vi "Motion@AddPallet__Parameter.vi"(1 "ParamterIn":string) -> (0 "ParamterOut":string)   [LabVIEW 2020]
panel:
  in  "AXIS":string(combo)
  in  "PointName":string(combo)
  in  "Speed":string(combo)
  in  "MotorName":string(combo)
  in  "Confirm":bool
  # "Motion@AddPallet $Motor,$Speed,$Point(@AXIS)\nExample:  $Point@XY will move XY only\n               $Point@XYZ(5) will move XYZ and Z will replace by 5"
  # "@"
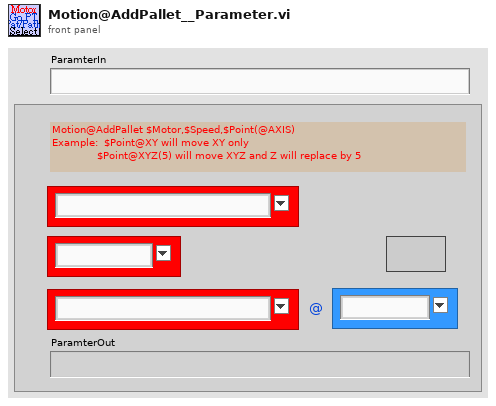
[diagram p1: front panel]
types:
  T1 = enum16{"Get", "UpdatePointS", "Init", "UpdateIndex", "GetCurrent&Index+1", "GetWithIndex", "ChkLast", "GetCurrent"}
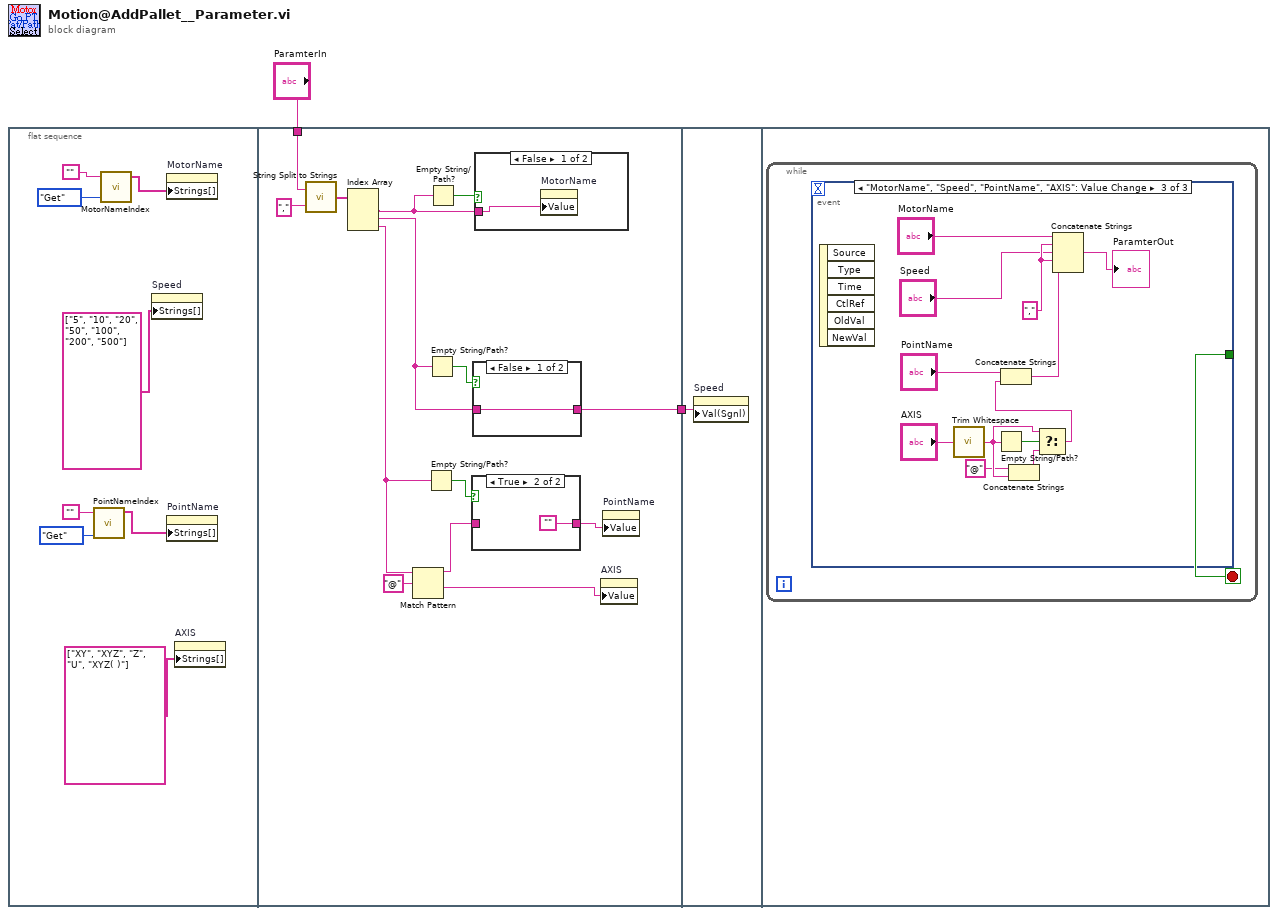
[diagram p0: block diagram]
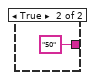
[diagram p3: hidden frame]
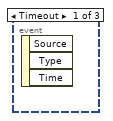
[diagram p5: hidden frame]
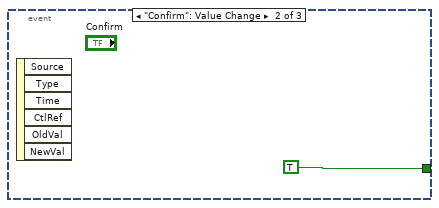
[diagram p6: hidden frame]
diagram:
  n1 = flat-sequence {
    tunnel: "ParamterIn" -> [w20]
    tunnel: [w16] -> w1
    tunnel: w1 -> [w30]
    frame #0 {
      n2 = call "PointNameIndex.vi"("OP"=T1."Get", "PointName"="") -> ("PointNameList"=w4:string[])  [unwired: 4 in, 5 out]
      n3 = call "MotorNameIndex.vi"("OP"=enum16{"Get", "Update", "Init"}."Get", "MotorName"="") -> ("MotorList"=w8:string[])  [unwired: 1 in, 2 out]
      n4 = property on="Speed" class="CmbBox"("Strings[]"=string[] ["5", "10", "20", "50", "100", "200", "500"] ("Strings []")) -> ()  [unwired: 2 in, 2 out]
      n5 = property on="MotorName" class="CmbBox"("Strings[]"=w8) -> ()  [unwired: 2 in, 2 out]
      n6 = property on="PointName" class="CmbBox"("Strings[]"=w4) -> ()  [unwired: 2 in, 2 out]
      n7 = property on="AXIS" class="CmbBox"("Strings[]"=string[] ["XY", "XYZ", "Z", "U", "XYZ( )"] ("Strings []")) -> ()  [unwired: 2 in, 2 out]
    }
    frame #1 {
      n8 = call "String Split to Strings.vi"("search string/char (-)"=",", "String"=w20) -> ("Array"=w22:string[])
      n9 = Index Array(array=w22) -> (element #1=w19:string, element #2=w18:string, element #3=w14:string)  [unwired: 3 in]
      n10 = Match Pattern(string=w14, regular expression="@") -> (before substring=w11:string, after substring=w12:string)  [unwired: 1 in, 2 out]
      n11 = Empty String/Path?(string/path=w14) -> (empty?=w17:bool)
      n12 = Empty String/Path?(string/path=w18) -> (empty?=w23:bool)
      n13 = Empty String/Path?(string/path=w19) -> (empty?=w24:bool)
      n14 = case shown="True" w17 {
        tunnel: [w25 ""] -> w15
        tunnel: w11 -> [w25 _]
        frame False {
        }
        frame True {
        }
      }
      n15 = case shown="False" w23 {
        tunnel: [w27 "50" ("ParamterIn")] -> w16
        tunnel: w18 -> [w27 _]
        frame False {
        }
        frame True {
        }
      }
      n16 = case shown="False" w24 {
        tunnel: w19 -> [w29 _]
        frame False {
          n17 = property on="MotorName" class="CmbBox"("Value"=w29) -> ()  [unwired: 2 in, 2 out]
        }
        frame True {
        }
      }
      n18 = property on="AXIS" class="CmbBox"("Value"=w12) -> ()  [unwired: 2 in, 2 out]
      n19 = property on="PointName" class="CmbBox"("Value"=w15) -> ()  [unwired: 2 in, 2 out]
    }
    frame #2 {
      n20 = property on="Speed" class="CmbBox"("Val(Sgnl)"=w30) -> ()  [unwired: 2 in, 2 out]
    }
    frame #3 {
      n21 = while {
        stop <- w31 stop-if-true
        n22 = event shown="[2] \"MotorName\", \"Speed\", \"PointName\", \"AXIS\": Value Change" {
          selector: _ -> [_ _ _]
          dyn-events: _ -> [_ _ _]
          timeout: _ -> [_ _ _]
          tunnel: [_ TRUE _] -> w31
          event Timeout {
            n23 = event-data() -> ()  [unwired: 1 in, 3 out]
          }
          event "Confirm": Value Change {
            n24 = event-data() -> ()  [unwired: 1 in, 6 out]
          }
          event "MotorName", "Speed", "PointName", "AXIS": Value Change {
            w42 = "," ("string")
            n25 = event-data() -> ()  [unwired: 1 in, 6 out]
            n26 = call <vilib>:"Trim Whitespace.vi"("string"="AXIS") -> ("trimmed string"=w37:string)  [unwired: 1 in]
            n27 = Empty String/Path?(string/path=w37) -> (empty?=w39:bool)
            n28 = Concatenate Strings("@" ("string"), w37) -> (w38:string)
            n29 = Select(t=w37, s=w39, f=w38) -> (s? t:f=w34:string)
            n30 = Concatenate Strings("PointName", w34) -> (w33:string)
            n31 = Concatenate Strings("MotorName", w42, "Speed", w42, w33) -> (→"ParamterOut":string)
          }
        }
      }
    }
  }
